vi "Ask Controller to Launch Results UI.vi"(8 "error in (no error)":errorcluster, 11 "Operator UI in":refnum<class "Controller UI.lvclass">) -> (0 "error out":errorcluster, 3 "Operator UI out":refnum<class "Controller UI.lvclass">)   [LabVIEW 2016, in "Controller UI.lvlib" / "Controller UI.lvclass"]
uses:
  <userlib>/Common Components/Controller UI/Controller UI.lvclass
  C:/Program Files (x86)/National Instruments/LabVIEW 2016/user.lib/Common Components/User Interface/UI.lvclass
  C:/Program Files (x86)/National Instruments/LabVIEW 2016/vi.lib/ActorFramework/Actor/Actor.lvclass
  <userlib>/Common Components/Controller UI/Controller UI.lvclass/Controller UI.ctl
  <vilib>/ActorFramework/Actor/Actor.lvclass/Actor.ctl
  <userlib>/Common Components/Controller/Messages/Launch Results UI Msg/Launch Results UI Msg.lvclass/Launch Results UI Msg.ctl
  <vilib>/ActorFramework/Message Enqueuer/Message Enqueuer.lvclass/Message Enqueuer.ctl
  <userlib>/Common Components/Controller UI/Accessors/Read Results Listbox.vi
  <vilib>/ActorFramework/Message Enqueuer/Enqueue.vi
  <userlib>/Common Components/Controller/Messages/Launch Results UI Msg/Launch Results UI Msg.lvclass
  C:/Program Files (x86)/National Instruments/LabVIEW 2016/vi.lib/ActorFramework/Message/Message.lvclass
  <vilib>/ActorFramework/Message Priority Queue/Priority Enqueue.vi
  <userlib>/Common Components/User Interface/UI.lvclass
  <vilib>/ActorFramework/Actor/Actor.lvclass
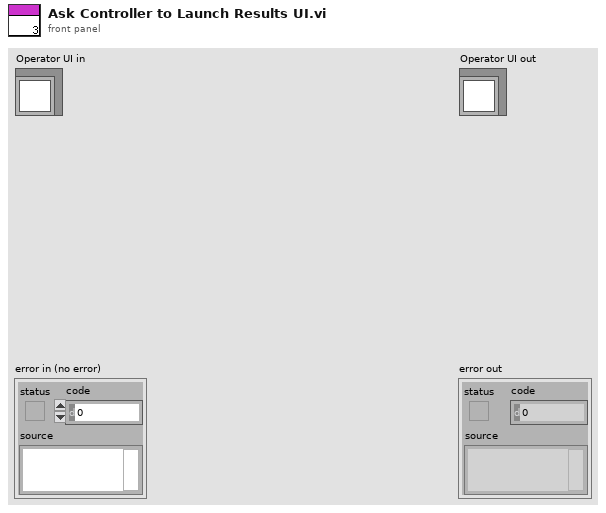
[diagram p1: front panel]
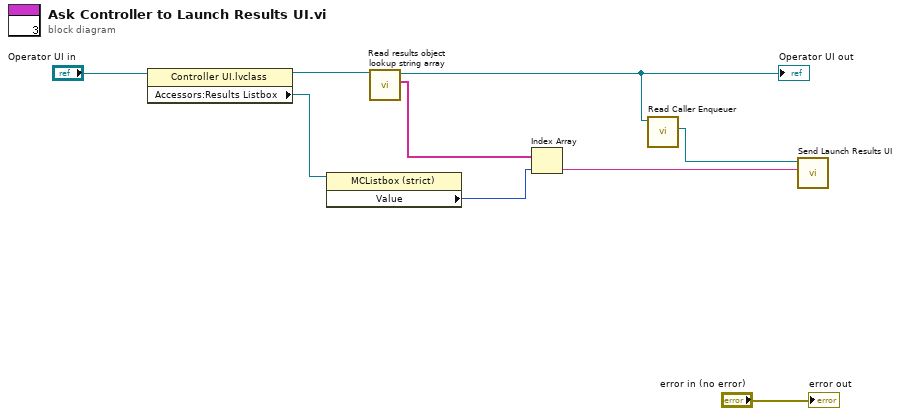
[diagram p0: block diagram]
diagram:
  n1 = property class="Controller UI.lvclass"(reference="Operator UI in") -> (reference out=w1:refnum<class "Controller UI.lvclass">, "Accessors:Results Listbox"=w2:refnum<vi>)  [unwired: 1 in, 1 out]
  n2 = property class="MCListbox (strict)"(reference=w2) -> ("Value"=w8:i32)  [unwired: 1 in, 2 out]
  n3 = call <userlib>:"Read results object lookup string array.vi"("UI in"=w1) -> ("results object lookup string array"=w7:string[], "UI out"=w5:refnum<class "Controller UI.lvclass">)  [unwired: 8 in, 1 out]
  "Operator UI out" <- w5
  n4 = Index Array(array=w7, index=w8) -> (element=w6:string)
  n5 = call <vilib>:"Read Caller Enqueuer.vi"("Actor"=w5) -> ("Caller Enqueuer"=w4:refnum<class "Message Enqueuer.lvclass">)  [unwired: 10 in]
  n6 = call <userlib>:"Send Launch Results UI.vi"("uniqueresultsid"=w6, "Message Enqueuer in"=w4) -> ()  [unwired: 8 in, 2 out]
  "error out" <- "error in (no error)"
